vi "R45_2-FPGA.vi"() -> ()   [LabVIEW 2016]
uses:
  control vi/controls/Aperture Readback.ctl
  control vi/controls/Faraday Cup Readback.ctl
  control vi/controls/Glassman Control.ctl
  control vi/controls/Glassman Readback.ctl
  <vilib>/LabVIEW Targets/FPGA/cRIO/shared/nicrio_ModuleControls/nicrio_cRIO-9871_BaudRateEnum.ctl
  <vilib>/LabVIEW Targets/FPGA/cRIO/shared/nicrio_ModuleControls/nicrio_cRIO-9871_DataBitsEnum.ctl
  <vilib>/LabVIEW Targets/FPGA/cRIO/shared/nicrio_ModuleControls/nicrio_cRIO-9871_ParityEnum.ctl
  <vilib>/LabVIEW Targets/FPGA/cRIO/shared/nicrio_ModuleControls/nicrio_cRIO-9871_StopBitsEnum.ctl
  <vilib>/Platform/TimedLoop/XDataNode/timing_clust.ctl
  <vilib>/Platform/TimedLoop/XDataNode/nitl_modes.ctl
  <vilib>/Platform/TimedLoop/XDataNode/wakeup.ctl
  <vilib>/rvi/FXPMathLib/basic elements/FxpIntAccumulator/subVIs/nifxpmath_IntAccumulator_SimConfig.ctl
  <vilib>/rvi/Emulation/niFpgaGetClockAttributes.vi
  <vilib>/rvi/Emulation/niFpgaSctlEmulationGetInTimedLoop.vi
  <vilib>/rvi/Emulation/niFpgaEmulationReportErrorSimple.vi
  <vilib>/rvi/eio/common/nirviEmuTemplateMethod_errors.vi
  <vilib>/rvi/Emulation/niFpgaCriticalErrorInLSC.vi
  <vilib>/rvi/Analysis/common/codeGenErrors/XNode/niFpgaXNodeCodeGenErrorHandle.vi
  <vilib>/rvi/FXPMathLib/basic elements/FxpIntAccumulator/simVIs/DllFxpIntAccumulator_sub.vi
  <vilib>/rvi/eio/common/nirviEmuTemplatePropertySet_errors.vi
  <vilib>/eio/EIONode/EIONode.xnode
  <vilib>/rvi/Analysis/measure/dc-rms/XNode/niFpgaDC-RMS.xnode
  <vilib>/Platform/TimedLoop/XDataNode/XDataNode.xnode
  <vilib>/rvi/FXPMathLib/basic elements/FxpIntAccumulator/XNode/nifxpmath_IntAccumulator.xnode
  <vilib>/rvi/FXPMathLib/FxpMul/XNode/nifxpmath_Multiplier.xnode
  <vilib>/eio/EIOPropertyNode/EIOPropertyNode.xnode
  <vilib>/eio/EIOMethodNode/EIOMethodNode.xnode
  <vilib>/Platform/TimedLoop/XDataNode/XDNodeRunTimeDep.lvlib
  <vilib>/rvi/FXPMathLib/sim/FxpSim.dll
  <vilib>/rvi/eio/common/nirviEmuTemplatePropertyGet_errors.vi
  <vilib>/rvi/eio/common/nirviEmuTemplatePropertyGet_noerrors.vi
  <vilib>/rvi/eio/common/nirviEmuTemplatePropertySet_noerrors.vi
panel:
  out "ExB 2- Monitor":T1
  out "ExB 2+ Monitor":T1
  out "ExB 1- Monitor":T1
  out "ExB 1+ Monitor":T1
  in  "ExB 2 - Voltage Set":T2
  in  "ExB 1 - Voltage Set":T2
  out "Detector FC Position":T3
  out "Detector Aperture Position":T4
  in  "Detector Aperture insert":bool
  out "ExB 2 PS error":errorcluster
  out "Position-Status Sensor error":errorcluster
  out "Cup-Aperture Control Loop Error":errorcluster
  in  "RT error":bool
  out "Vac Cluster 4 Ion Gauge 2":u8[](array[numeric])
  out "Vac Cluster 4 Convectron 2":u8[](array[numeric])
  out "Vac Cluster 4 Convectron 1":u8[](array[numeric])
  out "Vac Cluster 4 Ion Gauge 1":u8[](array[numeric])
  out "Vacuum Gauge 4 error":errorcluster
  out "Vac Cluster 3 Ion Gauge 2":u8[](array[numeric])
  out "Vac Cluster 3 Convectron 2":u8[](array[numeric])
  out "Vac Cluster 3 Convectron 1":u8[](array[numeric])
  out "Vac Cluster 3 Ion Gauge 1":u8[](array[numeric])
  out "Vacuum Gauge 3 error":errorcluster
  out "Vacuum Gauge 2 error":errorcluster
  out "GFM Hall Probe error":errorcluster
  out "GFM ps error":errorcluster
  out "ExB 1 PS error":errorcluster
  out "HV Control Loop error":errorcluster
  out "HV Readback Loop":errorcluster
  out "Hall Probe Data":u8
  out "Timed Out":bool
  out "GFM read":u8[](array[numeric])
  in  "GFM ps set":u8[](array[numeric])=[0, 0, 0, 0, 0, 0, 0, 0, 0, 0]
  in  "ExB 2 Reset":bool
  in  "ExB 2 PS set":u8[](array[numeric])=[0, 0, 0, 0, 0, 0, 0, 0, 0, 0]
  out "Vac Cluster 2 Ion Gauge 2":u8[](array[numeric])
  out "Vac Cluster 2 Convectron 2":u8[](array[numeric])
  out "Vac Cluster 2 Convectron 1":u8[](array[numeric])
  out "Vac Cluster 2 Ion Gauge 1":u8[](array[numeric])
  in  "ExB 1 PS set":u8[](array[numeric])=[0, 0, 0, 0, 0, 0, 0, 0, 0, 0]
  in  "Detector FC insert":bool
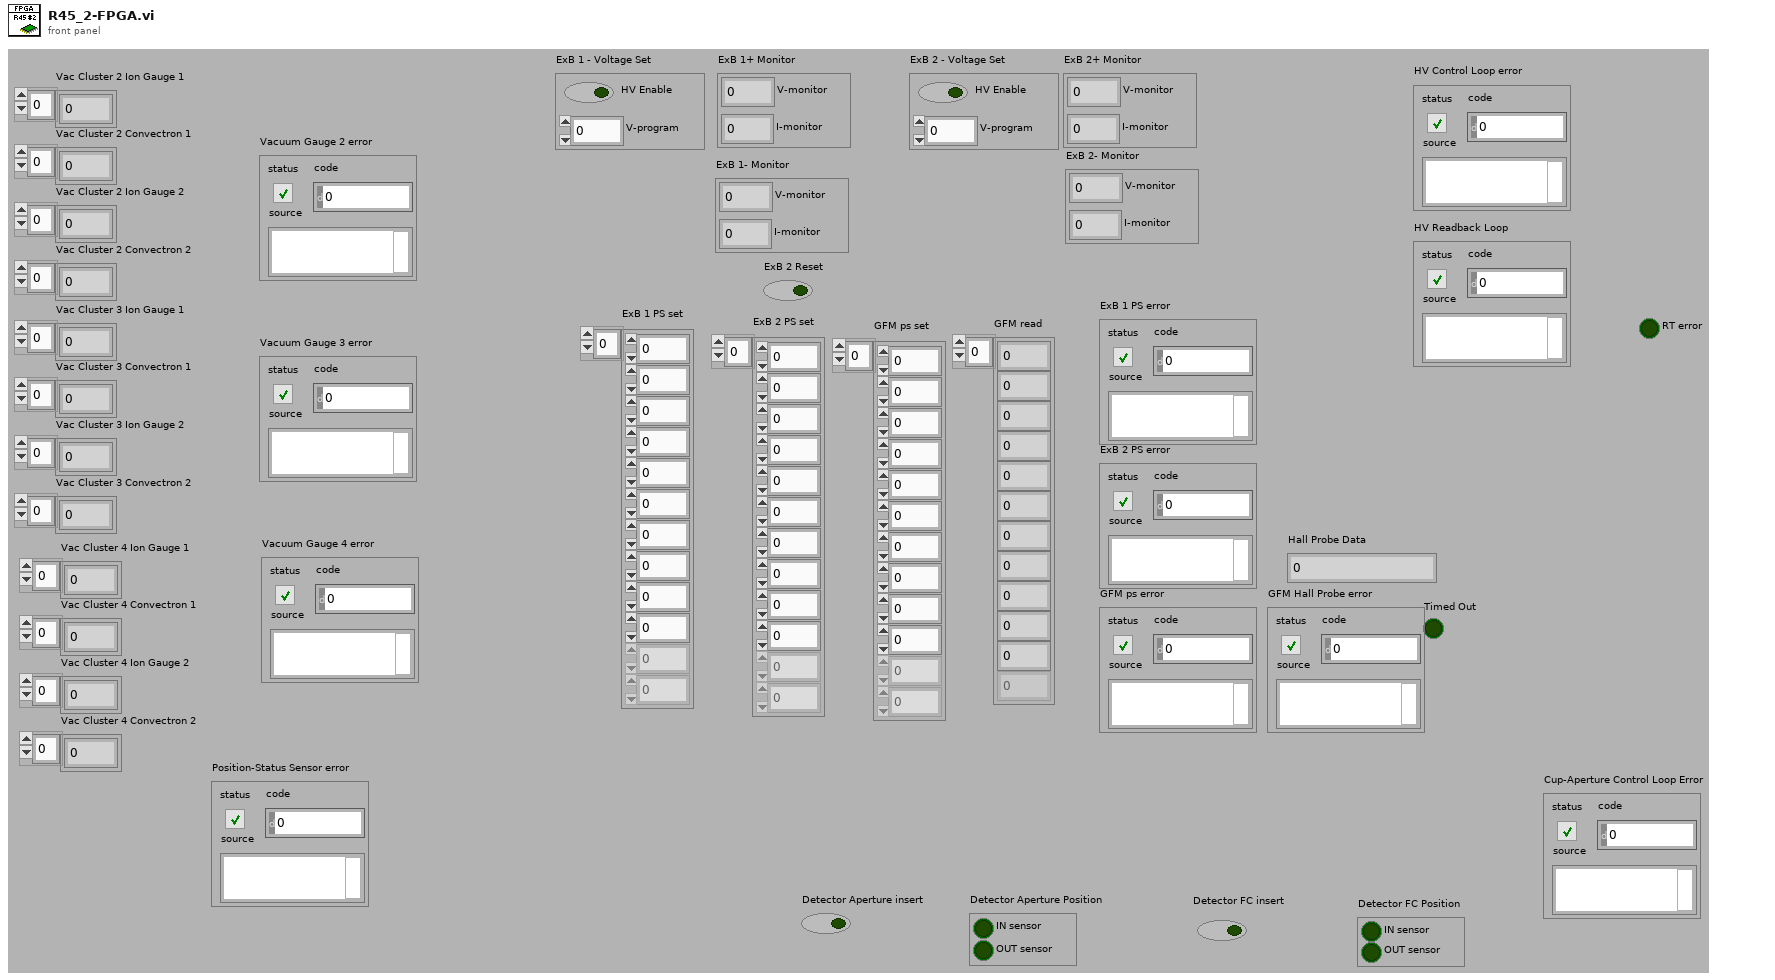
[diagram p1: front panel]
types:
  T1 = typedef "Glassman Readback.ctl" = cluster{"I-monitor":fxp<+/-,16,5>, "V-monitor":fxp<+/-,16,5>}
  T2 = typedef "Glassman Control.ctl" = cluster{"V-program":fxp<+/-,16,5>, "HV Enable":bool}
  T3 = typedef "Faraday Cup Readback.ctl" = cluster{"IN sensor":bool, "OUT sensor":bool}
  T4 = typedef "Aperture Readback.ctl" = cluster{"IN sensor":bool, "OUT sensor":bool}
  T5 = typedef "nicrio_cRIO-9871_StopBitsEnum.ctl" = enum8{"1", "1.5", "2"}
  T6 = typedef "nicrio_cRIO-9871_DataBitsEnum.ctl" = enum8{"5", "6", "7", "8"}
  T7 = typedef "nicrio_cRIO-9871_BaudRateEnum.ctl" = enum16{"75 bps", "110 bps", "134 bps", "150 bps", "300 bps", "600 bps", "1200 bps", "1800 bps", "2400 bps", "4800 bps", "7200 bps", "9600 bps", "14.4 kbps", "19.2 kbps", "28.8 kbps", "38.4 kbps", "57.6 kbps", "115.2 kbps", "230.4 kbps", "460.8 kbps", "921.6 kbps"}
  T8 = typedef "nicrio_cRIO-9871_ParityEnum.ctl" = enum8{"None", "Odd", "Even", "Mark", "Space"}
  T9 = typedef "XDNodeRunTimeDep.lvlib/timing_clust.ctl" = cluster{"Expected End [f-1]":u64, "Actual End [f-1]":u64, "Finished Late? [f-1]":bool, "Expected End [i-1]":u64, "Actual End [i-1]":u64, "Finished Late? [i-1]":bool, "Expected Start [i]":u64, "Actual Start [i]":u64, "Expected Start [f]":u64, "Actual Start [f]":u64, "Source Name":string, "Structure Name":string, "Period":i64, "Deadline":i64, "Offset":i64, "Start":i64, "Priority":i32, "Timeout":i32, "Mode":T10, "Wakeup Reason":T11, "Error":errorcluster, "Source Type":string, "Secondary Source Type":string, "Global End Time":u64, "Global Start Time":u64, "Frame Duration":u64, "Iteration Duration":u64, "Assigned CPU":i32, "I/O Scan Engine Mode":u32}
  T10 = typedef "XDNodeRunTimeDep.lvlib/nitl_modes.ctl" = enum32{"No Change", "Process missed periods, maintain original phase", "Discard missed periods, maintain original phase", "Process missed periods, ignore original phase", "Discard missed periods, ignore original phase"}
  T11 = typedef "XDNodeRunTimeDep.lvlib/wakeup.ctl" = enum32{"Normal", "Aborted", "Asynchronous wakeup", "Timing source error", "Timed loop error", "Timeout"}
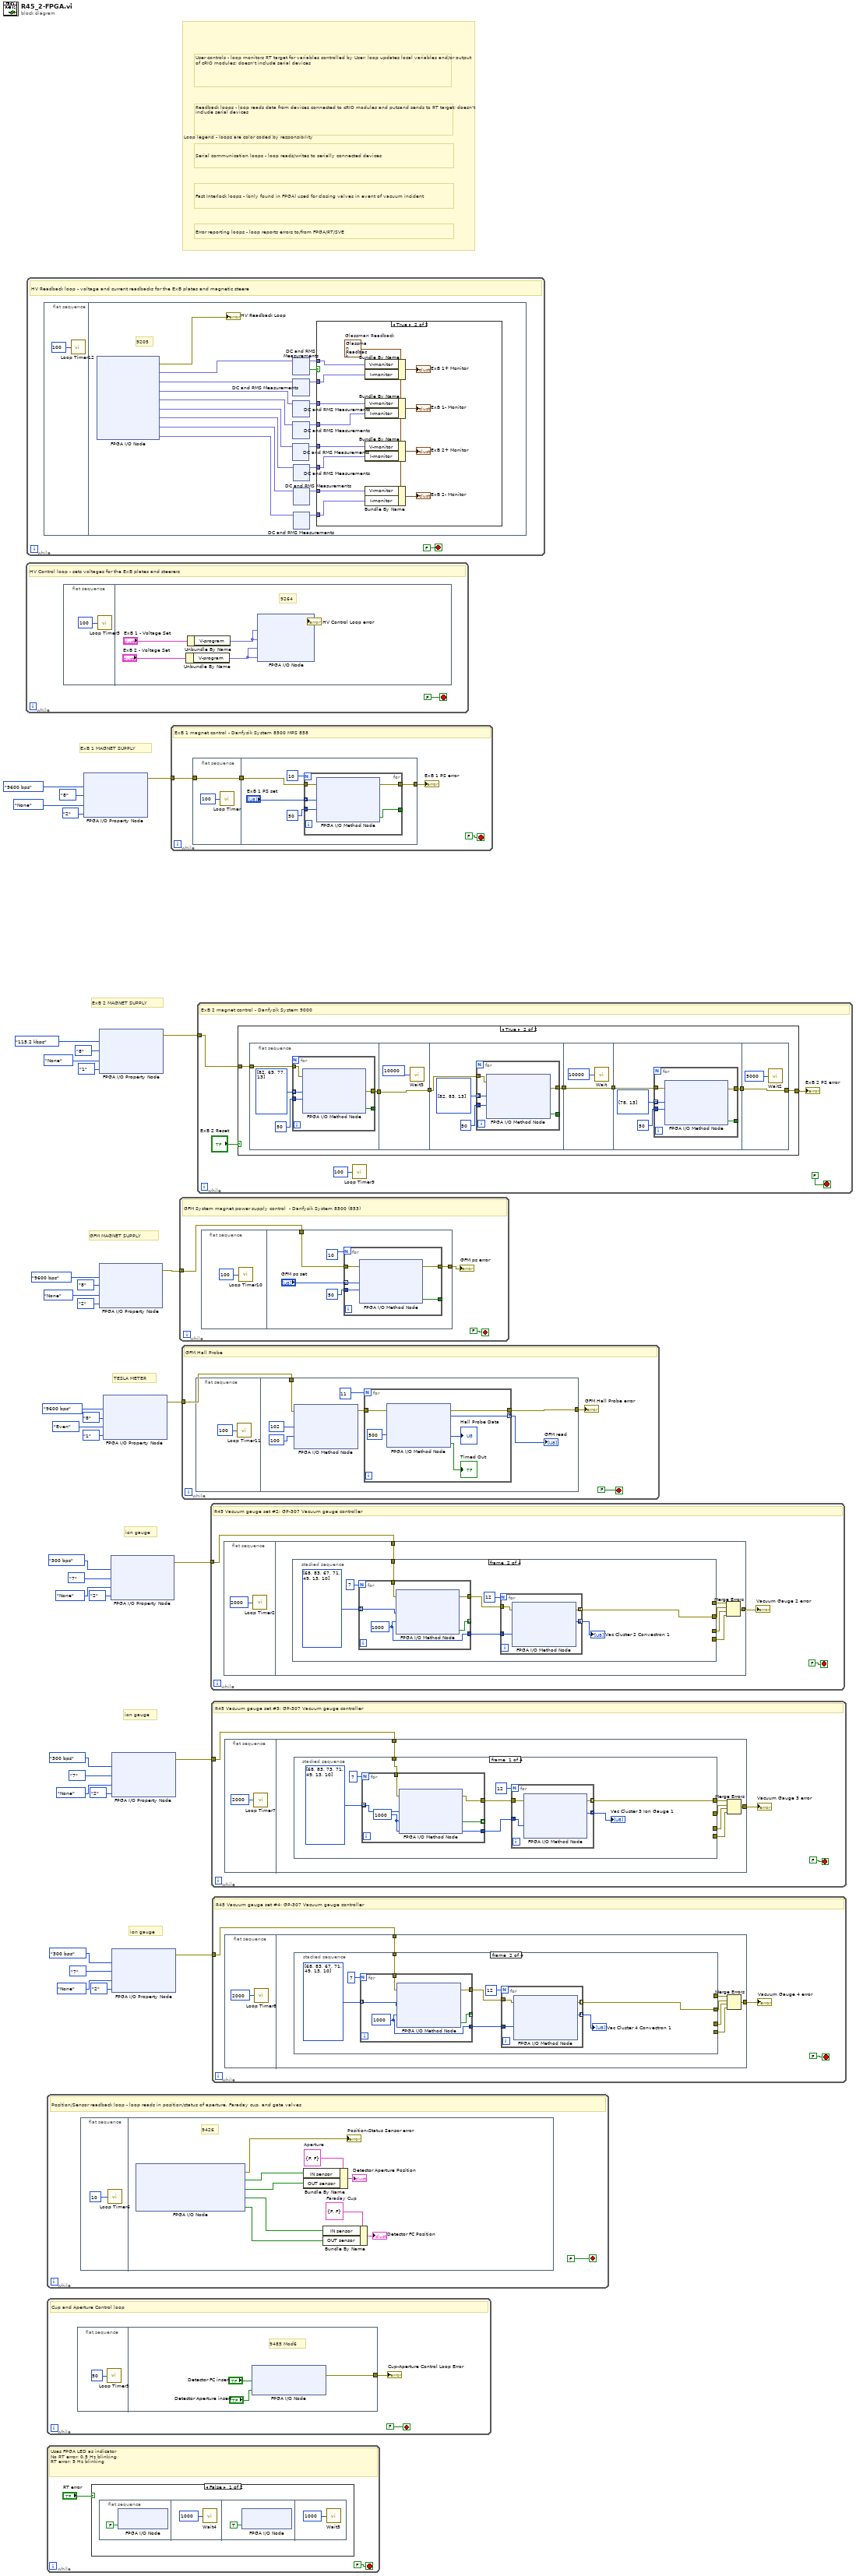
[diagram p0: block diagram]
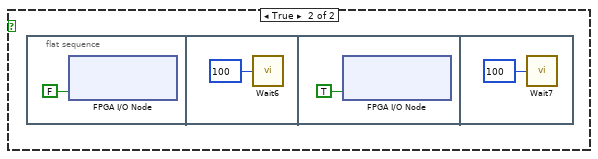
[diagram p2: hidden frame]
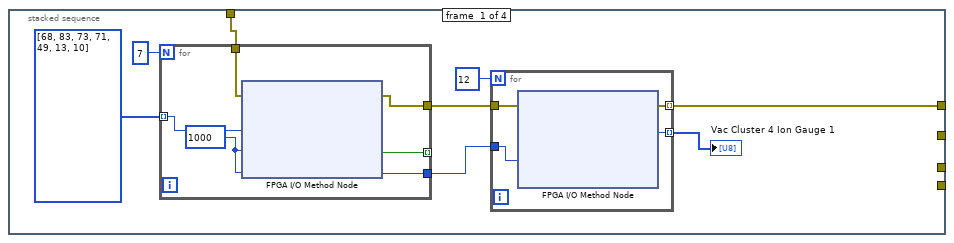
[diagram p3: hidden frame]
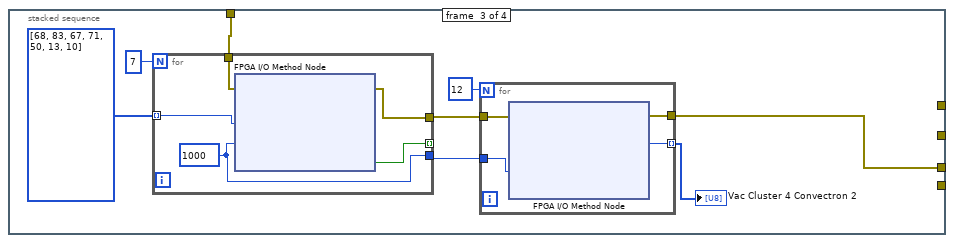
[diagram p4: hidden frame]
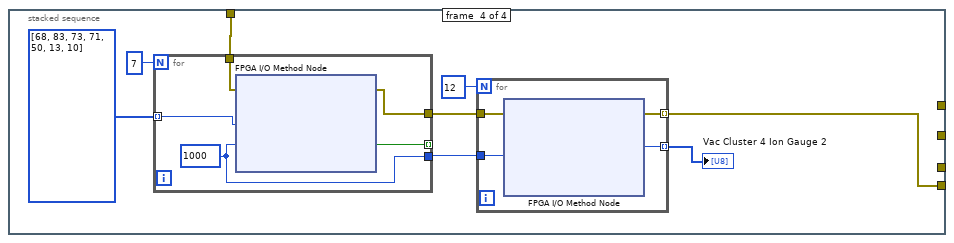
[diagram p5: hidden frame]
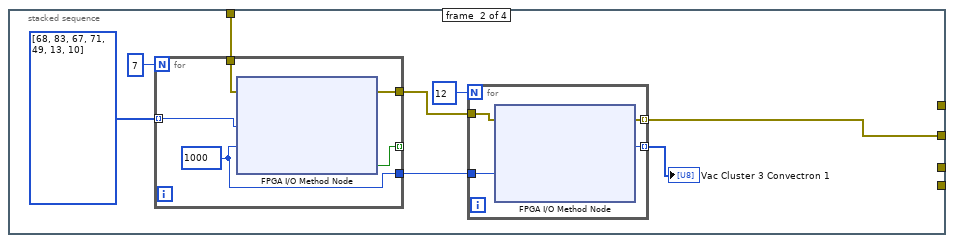
[diagram p6: hidden frame]
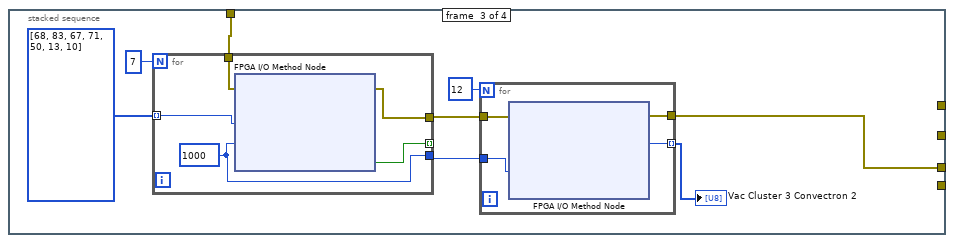
[diagram p7: hidden frame]
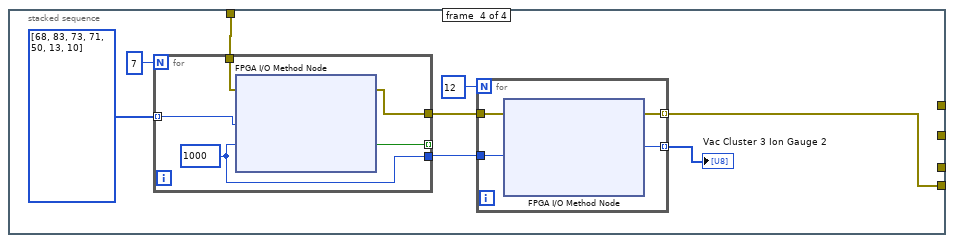
[diagram p8: hidden frame]
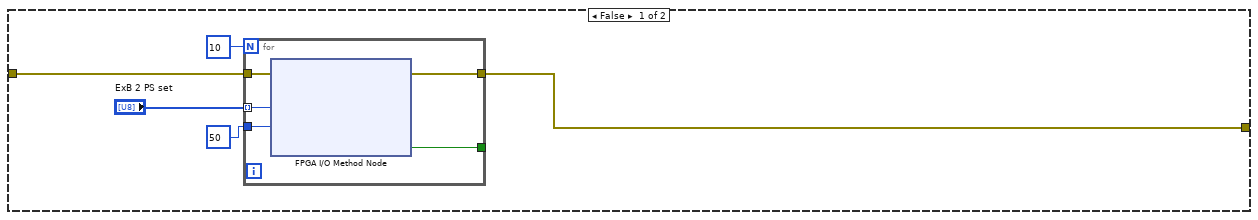
[diagram p10: hidden frame]
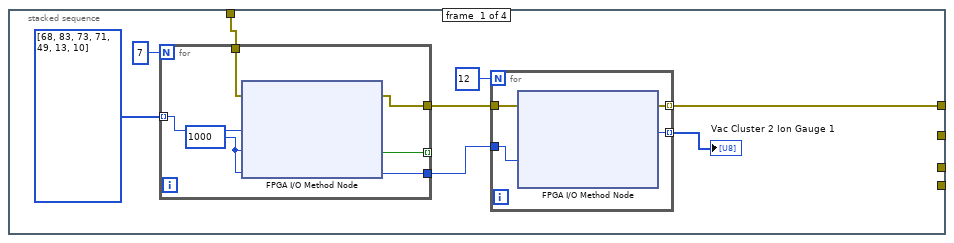
[diagram p11: hidden frame]
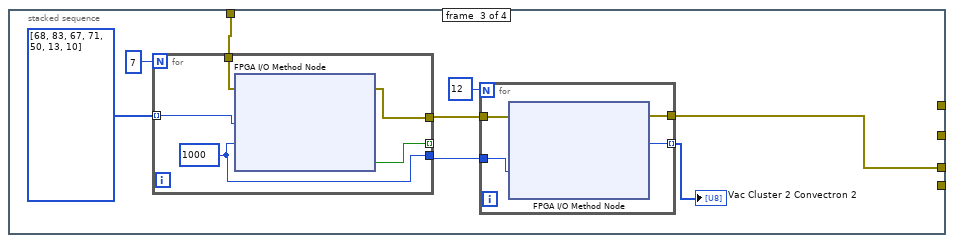
[diagram p12: hidden frame]
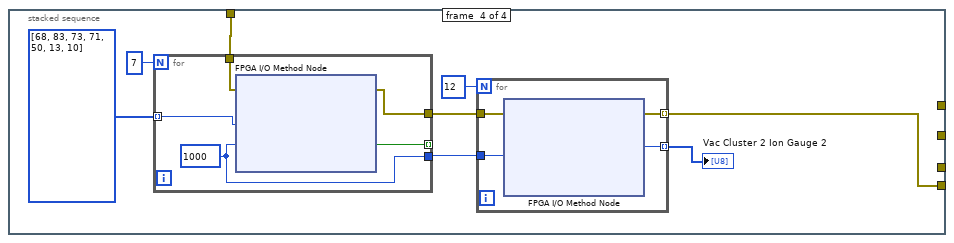
[diagram p13: hidden frame]
diagram:
  # "Fast Interlock loops - (only found in FPGA) used for closing valves in event of vacuum incident"
  # "Error reporting loops - loop reports errors to/from FPGA/RT/SVE"
  # "Serial communication loops - loop reads/writes to serially connected devices"
  # "Readback loops - loop reads data from devices connected to cRIO modules and putsand sends to RT target; doesn't include serial devices"
  # "User controls - loop monitors RT target for variables controlled by User; loop updates local variables and/or output of cRIO modules; doesn't include serial devices"
  # "Loop legend - loops are color coded by responsibility"
  # "TESLA METER"
  # "GFM MAGNET SUPPLY"
  # "ExB 2 MAGNET SUPPLY"
  # "ion gauge"
  # "ion gauge"
  # "ion gauge"
  # "ExB 1 MAGNET SUPPLY"
  n1 = while {
    stop <- FALSE stop-if-true
    # "HV Control loop - sets voltages for the ExB plates and steerers"
    n2 = flat-sequence {
      frame #0 {
        n3 = call "Loop Timer3"("Count(mSec)"=u32 100 ("Count(Ticks)")) -> ()  [unwired: 1 out]
      }
      frame #1 {
        # "9264"
        n4 = Unbundle By Name("ExB 2 - Voltage Set") -> ("V-program"=w39:fxp<+/-,16,5>)
        n5 = Unbundle By Name("ExB 1 - Voltage Set") -> ("V-program"=w40:fxp<+/-,16,5>)
        n6 = xnode "FPGA I/O Node"("ExB 1- V set"=w40, "ExB 1+ V set"=w40, "ExB 2- V set"=w39, "ExB 2+ V set"=w39) -> ("error out"=→"HV Control Loop error":errorcluster)  [unwired: 5 in, 4 out]
      }
    }
  }
  n7 = while {
    stop <- FALSE stop-if-true
    # "HV Readback loop - voltage and current readbacks for the ExB plates and magnetic steere"
    n8 = flat-sequence {
      frame #0 {
        n9 = call "Loop Timer12"("Count(mSec)"=u32 100 ("Count(Ticks)")) -> ()  [unwired: 1 out]
      }
      frame #1 {
        # "9205"
        n10 = xnode "FPGA I/O Node"() -> ("error out"=→"HV Readback Loop":errorcluster, "ExB 1+ V read"=w52:fxp<+/-,26,5>, "ExB 1+ I read"=w51:fxp<+/-,26,5>, "ExB 1- V read"=w50:fxp<+/-,26,5>, "ExB 1- I read"=w49:fxp<+/-,26,5>, "ExB 2+ V read"=w48:fxp<+/-,26,5>, "ExB 2+ I read"=w47:fxp<+/-,26,5>, "ExB 2- V read"=w46:fxp<+/-,26,5>, "ExB 2- I read"=w45:fxp<+/-,26,5>)  [unwired: 9 in, 8 out]
        n11 = xnode "DC and RMS Measurements"("input data"=w48) -> ("DC"=w57:fxp<+/-,26,5>)  [unwired: 1 in, 1 out]
        n12 = xnode "DC and RMS Measurements"("input data"=w52) -> ("DC"=w61:fxp<+/-,26,5>, "output valid"=w62:bool)  [unwired: 1 in]
        n13 = xnode "DC and RMS Measurements"("input data"=w51) -> ("DC"=w60:fxp<+/-,26,5>)  [unwired: 1 in, 1 out]
        n14 = xnode "DC and RMS Measurements"("input data"=w50) -> ("DC"=w59:fxp<+/-,26,5>)  [unwired: 1 in, 1 out]
        n15 = xnode "DC and RMS Measurements"("input data"=w49) -> ("DC"=w58:fxp<+/-,26,5>)  [unwired: 1 in, 1 out]
        n16 = xnode "DC and RMS Measurements"("input data"=w47) -> ("DC"=w56:fxp<+/-,26,5>)  [unwired: 1 in, 1 out]
        n17 = xnode "DC and RMS Measurements"("input data"=w46) -> ("DC"=w55:fxp<+/-,26,5>)  [unwired: 1 in, 1 out]
        n18 = xnode "DC and RMS Measurements"("input data"=w45) -> ("DC"=w54:fxp<+/-,26,5>)  [unwired: 1 in, 1 out]
        n19 = case shown="True" w62 {
          tunnel: w61 -> [_ w75]
          tunnel: w60 -> [_ w74]
          tunnel: w59 -> [_ w69]
          tunnel: w58 -> [_ w68]
          tunnel: w57 -> [_ w67]
          tunnel: w56 -> [_ w66]
          tunnel: w55 -> [_ w65]
          tunnel: w54 -> [_ w64]
          frame False {
          }
          frame True {
            w63 = T1 {"I-monitor"=0.0, "V-monitor"=0.0}  # Glassman Readback
            n20 = Bundle By Name(cluster=w63, "V-monitor"=w75, "I-monitor"=w74) -> (→"ExB 1+ Monitor":T1)
            n21 = Bundle By Name(cluster=w63, "V-monitor"=w69, "I-monitor"=w68) -> (→"ExB 1- Monitor":T1)
            n22 = Bundle By Name(cluster=w63, "V-monitor"=w67, "I-monitor"=w66) -> (→"ExB 2+ Monitor":T1)
            n23 = Bundle By Name(cluster=w63, "V-monitor"=w65, "I-monitor"=w64) -> (→"ExB 2- Monitor":T1)
          }
        }
      }
    }
  }
  n24 = while {
    stop <- FALSE stop-if-true
    # "Uses FPGA LED as indicator\nNo RT error: 0.5 Hz blinking\nRT error: 5 Hz blinking"
    n25 = case shown="False" "RT error" {
      frame False {
        n26 = flat-sequence {
          frame #0 {
            n27 = xnode "FPGA I/O Node"("FPGA LED"=FALSE) -> ()  [unwired: 1 in, 1 out]
          }
          frame #1 {
            n28 = call "Wait4"("Count(mSec)"=u16 1000) -> ()  [unwired: 1 out]
          }
          frame #2 {
            n29 = xnode "FPGA I/O Node"("FPGA LED"=TRUE) -> ()  [unwired: 1 in, 1 out]
          }
          frame #3 {
            n30 = call "Wait5"("Count(mSec)"=u16 1000) -> ()  [unwired: 1 out]
          }
        }
      }
      frame True {
        n31 = flat-sequence {
          frame #0 {
            n32 = xnode "FPGA I/O Node"("FPGA LED"=FALSE) -> ()  [unwired: 1 in, 1 out]
          }
          frame #1 {
            n33 = call "Wait6"("Count(mSec)"=u16 100) -> ()  [unwired: 1 out]
          }
          frame #2 {
            n34 = xnode "FPGA I/O Node"("FPGA LED"=TRUE) -> ()  [unwired: 1 in, 1 out]
          }
          frame #3 {
            n35 = call "Wait7"("Count(mSec)"=u16 100) -> ()  [unwired: 1 out]
          }
        }
      }
    }
  }
  n36 = while {
    stop <- FALSE stop-if-true
    # "Position/Sensor readback loop - loop reads in position/status of aperture, Faraday cup, and gate valves"
    n37 = flat-sequence {
      frame #0 {
        n38 = call "Loop Timer6"("Count(uSec)"=u32 10 ("Count(Ticks)")) -> ()  [unwired: 1 out]
      }
      frame #1 {
        w731 = T3 {"IN sensor"=FALSE, "OUT sensor"=FALSE}  # Faraday Cup
        w732 = T4 {"IN sensor"=FALSE, "OUT sensor"=FALSE}  # Aperture
        # "9426"
        n39 = xnode "FPGA I/O Node"() -> ("error out"=→"Position-Status Sensor error":errorcluster, "Detector Aperture IN sensor"=w734:bool, "Detector Aperture OUT sensor"=w733:bool, "Detector FC IN sensor"=w730:bool, "Detector FC OUT sensor"=w729:bool)  [unwired: 5 in, 4 out]
        n40 = Bundle By Name(cluster=w732, "IN sensor"=w734, "OUT sensor"=w733) -> (→"Detector Aperture Position":T4)
        n41 = Bundle By Name(cluster=w731, "IN sensor"=w730, "OUT sensor"=w729) -> (→"Detector FC Position":T3)
      }
    }
  }
  n42 = while {
    stop <- FALSE stop-if-true
    # "Cup and Aperture Control loop"
    n43 = flat-sequence {
      tunnel: [w741] -> w737
      frame #0 {
        n44 = call "Loop Timer5"("Count(mSec)"=u32 50 ("Count(Ticks)")) -> ()  [unwired: 1 out]
      }
      frame #1 {
        # "9485 Mod6"
        n45 = xnode "FPGA I/O Node"("Detector FC"="Detector FC insert", "Detector Aperture"="Detector Aperture insert") -> ("error out"=w741:errorcluster)  [unwired: 3 in, 2 out]
      }
    }
    "Cup-Aperture Control Loop Error" <- w737
  }
  n46 = xnode "FPGA I/O Property Node"("Baud Rate"=nicrio_cRIO-9871_BaudRateEnum."9600 bps", "Data Bits"=nicrio_cRIO-9871_DataBitsEnum."8", "Parity"=nicrio_cRIO-9871_ParityEnum."None", "Stop Bits"=nicrio_cRIO-9871_StopBitsEnum."2") -> ("error out"=w13:errorcluster)  [unwired: 2 in, 1 out]
  n47 = xnode "FPGA I/O Property Node"("Baud Rate"=nicrio_cRIO-9871_BaudRateEnum."9600 bps", "Data Bits"=nicrio_cRIO-9871_DataBitsEnum."8", "Parity"=nicrio_cRIO-9871_ParityEnum."None", "Stop Bits"=nicrio_cRIO-9871_StopBitsEnum."2") -> ("error out"=w8:errorcluster)  [unwired: 2 in, 1 out]
  n48 = xnode "FPGA I/O Property Node"("Baud Rate"=nicrio_cRIO-9871_BaudRateEnum."115.2 kbps", "Data Bits"=nicrio_cRIO-9871_DataBitsEnum."8", "Parity"=nicrio_cRIO-9871_ParityEnum."None", "Stop Bits"=nicrio_cRIO-9871_StopBitsEnum."1") -> ("error out"=w10:errorcluster)  [unwired: 2 in, 1 out]
  n49 = xnode "FPGA I/O Property Node"("Baud Rate"=nicrio_cRIO-9871_BaudRateEnum."9600 bps", "Data Bits"=nicrio_cRIO-9871_DataBitsEnum."8", "Parity"=nicrio_cRIO-9871_ParityEnum."Even", "Stop Bits"=nicrio_cRIO-9871_StopBitsEnum."1") -> ("error out"=w4:errorcluster)  [unwired: 2 in, 1 out]
  n50 = xnode "FPGA I/O Property Node"("Baud Rate"=nicrio_cRIO-9871_BaudRateEnum."300 bps", "Data Bits"=nicrio_cRIO-9871_DataBitsEnum."7", "Parity"=nicrio_cRIO-9871_ParityEnum."None", "Stop Bits"=nicrio_cRIO-9871_StopBitsEnum."2") -> ("error out"=w3:errorcluster)  [unwired: 2 in, 1 out]
  n51 = xnode "FPGA I/O Property Node"("Baud Rate"=nicrio_cRIO-9871_BaudRateEnum."300 bps", "Data Bits"=nicrio_cRIO-9871_DataBitsEnum."7", "Parity"=nicrio_cRIO-9871_ParityEnum."None", "Stop Bits"=nicrio_cRIO-9871_StopBitsEnum."2") -> ("error out"=w2:errorcluster)  [unwired: 2 in, 1 out]
  n52 = xnode "FPGA I/O Property Node"("Baud Rate"=nicrio_cRIO-9871_BaudRateEnum."300 bps", "Data Bits"=nicrio_cRIO-9871_DataBitsEnum."7", "Parity"=nicrio_cRIO-9871_ParityEnum."None", "Stop Bits"=nicrio_cRIO-9871_StopBitsEnum."2") -> ("error out"=w1:errorcluster)  [unwired: 2 in, 1 out]
  n53 = while {
    tunnel: w13 -> [w743]
    stop <- FALSE stop-if-true
    # "ExB 1 magnet control - Danfysik System 8500 MPS 858"
    n54 = flat-sequence {
      tunnel: [w747] -> w744
      tunnel: w743 -> [w747]
      tunnel: [w750] -> w745
      tunnel: w744 -> [w749]
      frame #0 {
        n55 = call "Loop Timer"("Count(mSec)"=u32 100) -> ()  [unwired: 1 out]
      }
      frame #1 {
        n56 = for {
          N: 10 -> [_]
          tunnel: 50 ("Timeout (ms)") -> [w758]
          tunnel: "ExB 1 PS set" -> [w757] mode=indexing
          tunnel: [w754] -> _
          tunnel: w749 -> [w756]
          tunnel: [w755] -> w750
          n57 = xnode "FPGA I/O Method Node"("error in"=w756, "Data"=w757, "Timeout (ms)"=w758) -> ("error out"=w755:errorcluster, "Timed Out"=w754:bool)  [unwired: 1 in, 1 out]
        }
      }
    }
    "ExB 1 PS error" <- w745
  }
  n58 = while {
    tunnel: w8 -> [w760]
    stop <- FALSE stop-if-true
    # "GFM System magnet power supply control  - Danfysik System 8500 (853)"
    n59 = flat-sequence {
      tunnel: w760 -> [w764]
      tunnel: [w763] -> w759
      frame #0 {
        n60 = call "Loop Timer10"("Count(mSec)"=u32 100) -> ()  [unwired: 1 out]
      }
      frame #1 {
        n61 = for {
          N: 10 -> [_]
          tunnel: 50 ("Timeout (ms)") -> [w769]
          tunnel: "GFM ps set" -> [w770] mode=indexing
          tunnel: w764 -> [w772]
          tunnel: [w771] -> w763
          tunnel: [w768] -> _
          n62 = xnode "FPGA I/O Method Node"("error in"=w772, "Data"=w770, "Timeout (ms)"=w769) -> ("error out"=w771:errorcluster, "Timed Out"=w768:bool)  [unwired: 1 in, 1 out]
        }
      }
    }
    "GFM ps error" <- w759
  }
  n63 = while {
    tunnel: w4 -> [w774]
    stop <- FALSE stop-if-true
    # "GFM Hall Probe"
    n64 = flat-sequence {
      tunnel: w774 -> [w780]
      tunnel: [w779] -> w773
      frame #0 {
        n65 = call "Loop Timer11"("Count(mSec)"=u32 100) -> ()  [unwired: 1 out]
      }
      frame #1 {
        n66 = xnode "FPGA I/O Method Node"("error in"=w780, "Data"=u8 102, "Timeout (ms)"=100) -> ("error out"=w781:errorcluster)  [unwired: 1 in, 2 out]
        n67 = for {
          N: 11 ("Numeric 3") -> [_]
          tunnel: [w787] -> w777 mode=indexing
          tunnel: w781 -> [w786]
          tunnel: [w785] -> w779
          n68 = xnode "FPGA I/O Method Node"("error in"=w786, "Timeout (ms)"=500) -> ("error out"=w785:errorcluster, "Data"=w787:u8, "Timed Out"=→"Timed Out":bool)  [unwired: 1 in, 1 out]
          "Hall Probe Data" <- w787
        }
        "GFM read" <- w777
      }
    }
    "GFM Hall Probe error" <- w773
  }
  n69 = while {
    tunnel: w10 -> [w790]
    stop <- FALSE stop-if-true
    # "ExB 2 magnet control - Danfysik System 9000"
    n70 = case shown="True" "ExB 2 Reset" {
      tunnel: w790 -> [w795 w810]
      tunnel: [w794 w804] -> w789
      frame False {
        n71 = for {
          N: 10 -> [_]
          tunnel: 50 ("Timeout (ms)") -> [w803]
          tunnel: "ExB 2 PS set" -> [w802] mode=indexing
          tunnel: [w801] -> _
          tunnel: w795 -> [w800]
          tunnel: [w799] -> w794
          n72 = xnode "FPGA I/O Method Node"("error in"=w800, "Data"=w802, "Timeout (ms)"=w803) -> ("error out"=w799:errorcluster, "Timed Out"=w801:bool)  [unwired: 1 in, 1 out]
        }
      }
      frame True {
        n73 = flat-sequence {
          tunnel: w810 -> [w812]
          tunnel: [w811] -> w808
          tunnel: [w820] -> w809
          tunnel: w808 -> [w820]
          tunnel: w809 -> [w823]
          tunnel: [w822] -> w806
          tunnel: [w831] -> w807
          tunnel: w806 -> [w831]
          tunnel: w807 -> [w834]
          tunnel: [w833] -> w805
          tunnel: w805 -> [w842]
          tunnel: [w842] -> w804
          frame #0 {
            n74 = for {
              tunnel: 50 ("Timeout (ms)") -> [w819]
              tunnel: u8[] [82, 69, 77, 13] ("unsigned byte array") -> [w818] mode=indexing
              tunnel: [w817] -> _
              tunnel: w812 -> [w816]
              tunnel: [w815] -> w811
              n75 = xnode "FPGA I/O Method Node"("error in"=w816, "Data"=w818, "Timeout (ms)"=w819) -> ("error out"=w815:errorcluster, "Timed Out"=w817:bool)  [unwired: 1 in, 1 out]
            }
          }
          frame #1 {
            n76 = call "Wait3"("Count(mSec)"=u32 10000) -> ()  [unwired: 1 out]
          }
          frame #2 {
            n77 = for {
              tunnel: 50 ("Timeout (ms)") -> [w830]
              tunnel: u8[] [82, 83, 13] ("unsigned byte array") -> [w829] mode=indexing
              tunnel: [w828] -> _
              tunnel: w823 -> [w826]
              tunnel: [w827] -> w822
              n78 = xnode "FPGA I/O Method Node"("error in"=w826, "Data"=w829, "Timeout (ms)"=w830) -> ("error out"=w827:errorcluster, "Timed Out"=w828:bool)  [unwired: 1 in, 1 out]
            }
          }
          frame #3 {
            n79 = call "Wait"("Count(mSec)"=u32 10000) -> ()  [unwired: 1 out]
          }
          frame #4 {
            n80 = for {
              tunnel: 50 ("Timeout (ms)") -> [w841]
              tunnel: u8[] [78, 13] ("unsigned byte array") -> [w840] mode=indexing
              tunnel: [w839] -> _
              tunnel: w834 -> [w838]
              tunnel: [w837] -> w833
              n81 = xnode "FPGA I/O Method Node"("error in"=w838, "Data"=w840, "Timeout (ms)"=w841) -> ("error out"=w837:errorcluster, "Timed Out"=w839:bool)  [unwired: 1 in, 1 out]
            }
          }
          frame #5 {
            n82 = call "Wait2"("Count(mSec)"=u32 5000) -> ()  [unwired: 1 out]
          }
        }
      }
    }
    "ExB 2 PS error" <- w789
    n83 = call "Loop Timer9"("Count(mSec)"=u32 100) -> ()  [unwired: 1 out]
  }
  n84 = while {
    tunnel: w3 -> [w845]
    stop <- FALSE stop-if-true
    # "R45 Vacuum gauge set #2: GP-307 Vacuum gauge controller"
    n85 = flat-sequence {
      tunnel: w845 -> [w853]
      tunnel: [w848] -> w844
      frame #0 {
        n86 = call "Loop Timer2"("Count(mSec)"=u32 2000 ("Count(Ticks)")) -> ()  [unwired: 1 out]
      }
      frame #1 {
        n87 = stacked-sequence {
          tunnel: [_ _ w890 _] -> w850
          tunnel: [_ _ _ w906] -> w849
          tunnel: w853 -> [w856 w873 w888 w905]
          tunnel: [w854 _ _ _] -> w852
          tunnel: [_ w872 _ _] -> w851
          frame #0 {
            n88 = for {
              N: 7 -> [_]
              tunnel: [w870] -> w857
              tunnel: [w869] -> _ mode=indexing
              tunnel: u8[] [68, 83, 73, 71, 49, 13, 10] ("unsigned byte array") -> [w868] mode=indexing
              tunnel: w856 -> [w867]
              tunnel: [w866] -> w855
              w870 = 1000 ("Timeout (ms)")
              n89 = xnode "FPGA I/O Method Node"("error in"=w867, "Data"=w868, "Timeout (ms)"=w870) -> ("error out"=w866:errorcluster, "Timed Out"=w869:bool)  [unwired: 1 in, 1 out]
            }
            n90 = for {
              N: 12 -> [_]
              tunnel: w857 -> [w865]
              tunnel: [w864] -> w858 mode=indexing
              tunnel: w855 -> [w863]
              tunnel: [w862] -> w854 mode=indexing
              n91 = xnode "FPGA I/O Method Node"("error in"=w863, "Timeout (ms)"=w865) -> ("error out"=w862:errorcluster, "Data"=w864:u8)  [unwired: 1 in, 2 out]
            }
            "Vac Cluster 2 Ion Gauge 1" <- w858
          }
          frame #1 {
            n92 = for {
              N: 7 -> [_]
              tunnel: [w886] -> w878
              tunnel: [w885] -> _ mode=indexing
              tunnel: u8[] [68, 83, 67, 71, 49, 13, 10] ("unsigned byte array") -> [w887] mode=indexing
              tunnel: w873 -> [w884]
              tunnel: [w883] -> w871
              w886 = 1000 ("Timeout (ms)")
              n93 = xnode "FPGA I/O Method Node"("error in"=w884, "Data"=w887, "Timeout (ms)"=w886) -> ("error out"=w883:errorcluster, "Timed Out"=w885:bool)  [unwired: 1 in, 1 out]
            }
            n94 = for {
              N: 12 -> [_]
              tunnel: w878 -> [w882]
              tunnel: [w881] -> w874 mode=indexing
              tunnel: w871 -> [w880]
              tunnel: [w879] -> w872 mode=indexing
              n95 = xnode "FPGA I/O Method Node"("error in"=w880, "Timeout (ms)"=w882) -> ("error out"=w879:errorcluster, "Data"=w881:u8)  [unwired: 1 in, 2 out]
            }
            "Vac Cluster 2 Convectron 1" <- w874
          }
          frame #2 {
            n96 = for {
              N: 7 -> [_]
              tunnel: [w902] -> w895
              tunnel: [w903] -> _ mode=indexing
              tunnel: u8[] [68, 83, 67, 71, 50, 13, 10] ("unsigned byte array") -> [w904] mode=indexing
              tunnel: [w901] -> w891
              tunnel: w888 -> [w900]
              w902 = 1000 ("Timeout (ms)")
              n97 = xnode "FPGA I/O Method Node"("error in"=w900, "Data"=w904, "Timeout (ms)"=w902) -> ("error out"=w901:errorcluster, "Timed Out"=w903:bool)  [unwired: 1 in, 1 out]
            }
            n98 = for {
              N: 12 -> [_]
              tunnel: w895 -> [w899]
              tunnel: [w898] -> w889 mode=indexing
              tunnel: w891 -> [w897]
              tunnel: [w896] -> w890
              n99 = xnode "FPGA I/O Method Node"("error in"=w897, "Timeout (ms)"=w899) -> ("error out"=w896:errorcluster, "Data"=w898:u8)  [unwired: 1 in, 2 out]
            }
            "Vac Cluster 2 Convectron 2" <- w889
          }
          frame #3 {
            n100 = for {
              N: 7 -> [_]
              tunnel: [w919] -> w912
              tunnel: [w921] -> _ mode=indexing
              tunnel: u8[] [68, 83, 73, 71, 50, 13, 10] ("unsigned byte array") -> [w920] mode=indexing
              tunnel: [w918] -> w907
              tunnel: w905 -> [w917]
              w919 = 1000 ("Timeout (ms)")
              n101 = xnode "FPGA I/O Method Node"("error in"=w917, "Data"=w920, "Timeout (ms)"=w919) -> ("error out"=w918:errorcluster, "Timed Out"=w921:bool)  [unwired: 1 in, 1 out]
            }
            n102 = for {
              N: 12 -> [_]
              tunnel: w912 -> [w916]
              tunnel: [w915] -> w908 mode=indexing
              tunnel: w907 -> [w914]
              tunnel: [w913] -> w906 mode=indexing
              n103 = xnode "FPGA I/O Method Node"("error in"=w914, "Timeout (ms)"=w916) -> ("error out"=w913:errorcluster, "Data"=w915:u8)  [unwired: 1 in, 2 out]
            }
            "Vac Cluster 2 Ion Gauge 2" <- w908
          }
        }
        n104 = Merge Errors(w852, w851, w850, w849) -> (w848:errorcluster)
      }
    }
    "Vacuum Gauge 2 error" <- w844
  }
  n105 = while {
    tunnel: w2 -> [w923]
    stop <- FALSE stop-if-true
    # "R45 Vacuum gauge set #3: GP-307 Vacuum gauge controller"
    n106 = flat-sequence {
      tunnel: w923 -> [w931]
      tunnel: [w926] -> w922
      frame #0 {
        n107 = call "Loop Timer7"("Count(mSec)"=u32 2000 ("Count(Ticks)")) -> ()  [unwired: 1 out]
      }
      frame #1 {
        n108 = stacked-sequence {
          tunnel: [_ _ w968 _] -> w928
          tunnel: [_ _ _ w984] -> w927
          tunnel: w931 -> [w934 w951 w966 w983]
          tunnel: [w932 _ _ _] -> w930
          tunnel: [_ w950 _ _] -> w929
          frame #0 {
            n109 = for {
              N: 7 -> [_]
              tunnel: [w948] -> w935
              tunnel: [w947] -> _ mode=indexing
              tunnel: u8[] [68, 83, 73, 71, 49, 13, 10] ("unsigned byte array") -> [w946] mode=indexing
              tunnel: w934 -> [w945]
              tunnel: [w944] -> w933
              w948 = 1000 ("Timeout (ms)")
              n110 = xnode "FPGA I/O Method Node"("error in"=w945, "Data"=w946, "Timeout (ms)"=w948) -> ("error out"=w944:errorcluster, "Timed Out"=w947:bool)  [unwired: 1 in, 1 out]
            }
            n111 = for {
              N: 12 -> [_]
              tunnel: w935 -> [w943]
              tunnel: [w942] -> w936 mode=indexing
              tunnel: w933 -> [w941]
              tunnel: [w940] -> w932 mode=indexing
              n112 = xnode "FPGA I/O Method Node"("error in"=w941, "Timeout (ms)"=w943) -> ("error out"=w940:errorcluster, "Data"=w942:u8)  [unwired: 1 in, 2 out]
            }
            "Vac Cluster 3 Ion Gauge 1" <- w936
          }
          frame #1 {
            n113 = for {
              N: 7 -> [_]
              tunnel: [w964] -> w956
              tunnel: [w963] -> _ mode=indexing
              tunnel: u8[] [68, 83, 67, 71, 49, 13, 10] ("unsigned byte array") -> [w965] mode=indexing
              tunnel: w951 -> [w962]
              tunnel: [w961] -> w949
              w964 = 1000 ("Timeout (ms)")
              n114 = xnode "FPGA I/O Method Node"("error in"=w962, "Data"=w965, "Timeout (ms)"=w964) -> ("error out"=w961:errorcluster, "Timed Out"=w963:bool)  [unwired: 1 in, 1 out]
            }
            n115 = for {
              N: 12 -> [_]
              tunnel: w956 -> [w960]
              tunnel: [w959] -> w952 mode=indexing
              tunnel: w949 -> [w958]
              tunnel: [w957] -> w950 mode=indexing
              n116 = xnode "FPGA I/O Method Node"("error in"=w958, "Timeout (ms)"=w960) -> ("error out"=w957:errorcluster, "Data"=w959:u8)  [unwired: 1 in, 2 out]
            }
            "Vac Cluster 3 Convectron 1" <- w952
          }
          frame #2 {
            n117 = for {
              N: 7 -> [_]
              tunnel: [w980] -> w973
              tunnel: [w981] -> _ mode=indexing
              tunnel: u8[] [68, 83, 67, 71, 50, 13, 10] ("unsigned byte array") -> [w982] mode=indexing
              tunnel: [w979] -> w969
              tunnel: w966 -> [w978]
              w980 = 1000 ("Timeout (ms)")
              n118 = xnode "FPGA I/O Method Node"("error in"=w978, "Data"=w982, "Timeout (ms)"=w980) -> ("error out"=w979:errorcluster, "Timed Out"=w981:bool)  [unwired: 1 in, 1 out]
            }
            n119 = for {
              N: 12 -> [_]
              tunnel: w973 -> [w977]
              tunnel: [w976] -> w967 mode=indexing
              tunnel: w969 -> [w975]
              tunnel: [w974] -> w968
              n120 = xnode "FPGA I/O Method Node"("error in"=w975, "Timeout (ms)"=w977) -> ("error out"=w974:errorcluster, "Data"=w976:u8)  [unwired: 1 in, 2 out]
            }
            "Vac Cluster 3 Convectron 2" <- w967
          }
          frame #3 {
            n121 = for {
              N: 7 -> [_]
              tunnel: [w997] -> w990
              tunnel: [w999] -> _ mode=indexing
              tunnel: u8[] [68, 83, 73, 71, 50, 13, 10] ("unsigned byte array") -> [w998] mode=indexing
              tunnel: [w996] -> w985
              tunnel: w983 -> [w995]
              w997 = 1000 ("Timeout (ms)")
              n122 = xnode "FPGA I/O Method Node"("error in"=w995, "Data"=w998, "Timeout (ms)"=w997) -> ("error out"=w996:errorcluster, "Timed Out"=w999:bool)  [unwired: 1 in, 1 out]
            }
            n123 = for {
              N: 12 -> [_]
              tunnel: w990 -> [w994]
              tunnel: [w993] -> w986 mode=indexing
              tunnel: w985 -> [w992]
              tunnel: [w991] -> w984 mode=indexing
              n124 = xnode "FPGA I/O Method Node"("error in"=w992, "Timeout (ms)"=w994) -> ("error out"=w991:errorcluster, "Data"=w993:u8)  [unwired: 1 in, 2 out]
            }
            "Vac Cluster 3 Ion Gauge 2" <- w986
          }
        }
        n125 = Merge Errors(w930, w929, w928, w927) -> (w926:errorcluster)
      }
    }
    "Vacuum Gauge 3 error" <- w922
  }
  n126 = while {
    tunnel: w1 -> [w1001]
    stop <- FALSE stop-if-true
    # "R45 Vacuum gauge set #4: GP-307 Vacuum gauge controller"
    n127 = flat-sequence {
      tunnel: w1001 -> [w1009]
      tunnel: [w1004] -> w1000
      frame #0 {
        n128 = call "Loop Timer8"("Count(mSec)"=u32 2000 ("Count(Ticks)")) -> ()  [unwired: 1 out]
      }
      frame #1 {
        n129 = stacked-sequence {
          tunnel: [_ _ w1046 _] -> w1006
          tunnel: [_ _ _ w1062] -> w1005
          tunnel: w1009 -> [w1012 w1029 w1044 w1061]
          tunnel: [w1010 _ _ _] -> w1008
          tunnel: [_ w1028 _ _] -> w1007
          frame #0 {
            n130 = for {
              N: 7 -> [_]
              tunnel: [w1026] -> w1013
              tunnel: [w1025] -> _ mode=indexing
              tunnel: u8[] [68, 83, 73, 71, 49, 13, 10] ("unsigned byte array") -> [w1024] mode=indexing
              tunnel: w1012 -> [w1023]
              tunnel: [w1022] -> w1011
              w1026 = 1000 ("Timeout (ms)")
              n131 = xnode "FPGA I/O Method Node"("error in"=w1023, "Data"=w1024, "Timeout (ms)"=w1026) -> ("error out"=w1022:errorcluster, "Timed Out"=w1025:bool)  [unwired: 1 in, 1 out]
            }
            n132 = for {
              N: 12 -> [_]
              tunnel: w1013 -> [w1021]
              tunnel: [w1020] -> w1014 mode=indexing
              tunnel: w1011 -> [w1019]
              tunnel: [w1018] -> w1010 mode=indexing
              n133 = xnode "FPGA I/O Method Node"("error in"=w1019, "Timeout (ms)"=w1021) -> ("error out"=w1018:errorcluster, "Data"=w1020:u8)  [unwired: 1 in, 2 out]
            }
            "Vac Cluster 4 Ion Gauge 1" <- w1014
          }
          frame #1 {
            n134 = for {
              N: 7 -> [_]
              tunnel: [w1042] -> w1034
              tunnel: [w1041] -> _ mode=indexing
              tunnel: u8[] [68, 83, 67, 71, 49, 13, 10] ("unsigned byte array") -> [w1043] mode=indexing
              tunnel: w1029 -> [w1040]
              tunnel: [w1039] -> w1027
              w1042 = 1000 ("Timeout (ms)")
              n135 = xnode "FPGA I/O Method Node"("error in"=w1040, "Data"=w1043, "Timeout (ms)"=w1042) -> ("error out"=w1039:errorcluster, "Timed Out"=w1041:bool)  [unwired: 1 in, 1 out]
            }
            n136 = for {
              N: 12 -> [_]
              tunnel: w1034 -> [w1038]
              tunnel: [w1037] -> w1030 mode=indexing
              tunnel: w1027 -> [w1036]
              tunnel: [w1035] -> w1028 mode=indexing
              n137 = xnode "FPGA I/O Method Node"("error in"=w1036, "Timeout (ms)"=w1038) -> ("error out"=w1035:errorcluster, "Data"=w1037:u8)  [unwired: 1 in, 2 out]
            }
            "Vac Cluster 4 Convectron 1" <- w1030
          }
          frame #2 {
            n138 = for {
              N: 7 -> [_]
              tunnel: [w1058] -> w1051
              tunnel: [w1059] -> _ mode=indexing
              tunnel: u8[] [68, 83, 67, 71, 50, 13, 10] ("unsigned byte array") -> [w1060] mode=indexing
              tunnel: [w1057] -> w1047
              tunnel: w1044 -> [w1056]
              w1058 = 1000 ("Timeout (ms)")
              n139 = xnode "FPGA I/O Method Node"("error in"=w1056, "Data"=w1060, "Timeout (ms)"=w1058) -> ("error out"=w1057:errorcluster, "Timed Out"=w1059:bool)  [unwired: 1 in, 1 out]
            }
            n140 = for {
              N: 12 -> [_]
              tunnel: w1051 -> [w1055]
              tunnel: [w1054] -> w1045 mode=indexing
              tunnel: w1047 -> [w1053]
              tunnel: [w1052] -> w1046
              n141 = xnode "FPGA I/O Method Node"("error in"=w1053, "Timeout (ms)"=w1055) -> ("error out"=w1052:errorcluster, "Data"=w1054:u8)  [unwired: 1 in, 2 out]
            }
            "Vac Cluster 4 Convectron 2" <- w1045
          }
          frame #3 {
            n142 = for {
              N: 7 -> [_]
              tunnel: [w1075] -> w1068
              tunnel: [w1077] -> _ mode=indexing
              tunnel: u8[] [68, 83, 73, 71, 50, 13, 10] ("unsigned byte array") -> [w1076] mode=indexing
              tunnel: [w1074] -> w1063
              tunnel: w1061 -> [w1073]
              w1075 = 1000 ("Timeout (ms)")
              n143 = xnode "FPGA I/O Method Node"("error in"=w1073, "Data"=w1076, "Timeout (ms)"=w1075) -> ("error out"=w1074:errorcluster, "Timed Out"=w1077:bool)  [unwired: 1 in, 1 out]
            }
            n144 = for {
              N: 12 -> [_]
              tunnel: w1068 -> [w1072]
              tunnel: [w1071] -> w1064 mode=indexing
              tunnel: w1063 -> [w1070]
              tunnel: [w1069] -> w1062 mode=indexing
              n145 = xnode "FPGA I/O Method Node"("error in"=w1070, "Timeout (ms)"=w1072) -> ("error out"=w1069:errorcluster, "Data"=w1071:u8)  [unwired: 1 in, 2 out]
            }
            "Vac Cluster 4 Ion Gauge 2" <- w1064
          }
        }
        n146 = Merge Errors(w1008, w1007, w1006, w1005) -> (w1004:errorcluster)
      }
    }
    "Vacuum Gauge 4 error" <- w1000
  }
